vi "SalcompMESCheck Process.vi"(5 "SN":string, 11 "错误输入（无错误）":errorcluster) -> (6 "Message":string, 10 "CheckRouteForSerialNumber":bool, 15 "错误输出":errorcluster)   [LabVIEW 2018]
uses:
  CMESAPI.dll
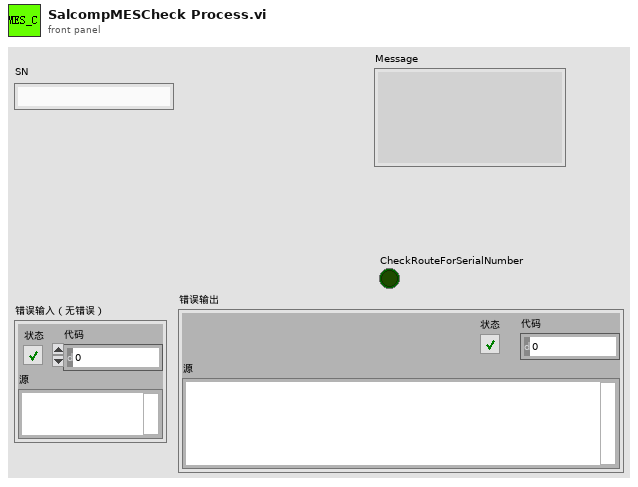
[diagram p1: front panel]
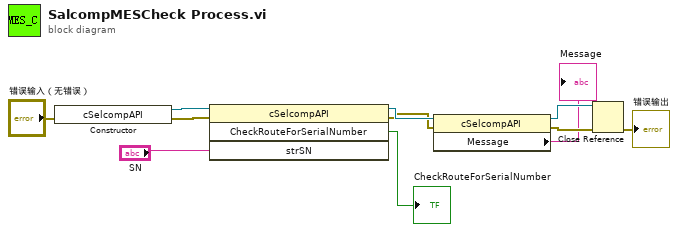
[diagram p0: block diagram]
diagram:
  n1 = constructor class="cSelcompAPI"(error in="错误输入（无错误）") -> (reference out=w11:refnum<k24>, error out=w10:errorcluster)  [unwired: 2 in, 1 out]
  n2 = invoke class="cSelcompAPI" method="CheckRouteForSerialNumber"(reference=w11, error in=w10, "strSN"="SN") -> (reference out=w9:refnum<k24>, error out=w8:errorcluster, "CheckRouteForSerialNumber"=→"CheckRouteForSerialNumber":bool)  [unwired: 1 in, 1 out]
  n3 = property class="cSelcompAPI"(reference=w9, error in=w8) -> (reference out=w7:refnum<k24>, error out=w6:errorcluster, "Message"=→"Message":string)
  n4 = Close Reference(reference=w7, error in (no error)=w6) -> (error out=→"错误输出":errorcluster)
